vi "Constants.vi"() -> ()   [LabVIEW 2017, in "Routing and Faulting Shared.lvlib"]
doc: "Use this Global VI to access the GUIDs assigned to the page resources of the Custom Device."
uses:
  Routing and Faulting Shared.lvlib
panel:
  in  "Tab Control":enum32{"GUIDS", "Constants", "Properties"}(tab)
  in  "Switching":string="ce8870b5-cb8e-4b52-ac34-5b792fdc2ead"
  in  "Aliases":string="58f3342d-82ee-4932-869a-6f49da3049e5"
  in  "Routing and Faulting":string="4e591626-626d-4903-9a6e-1f2a7b879f4d"
  in  "Compiled.Settings":string="Compiled.Settings"
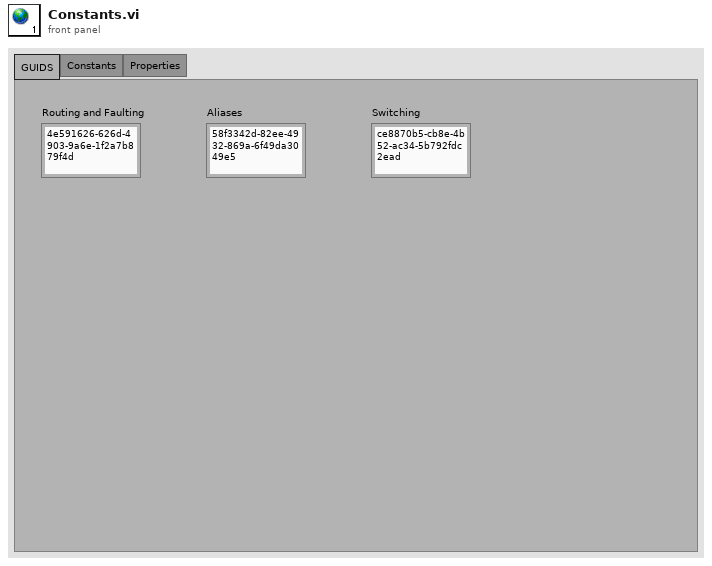
[diagram p1: front panel]
diagram:
